vi "readQPD3axissignal.vi"(9 "error out":errorcluster, 10 "Samples per Channel":i32, 11 "task in":refnum<k21>) -> (1 "X mean":dbl, 2 "Y mean":dbl, 3 "Z mean":dbl)   [LabVIEW 2014]
doc: "Read QPD 3 axis signal according to the input DAQ task."
uses:
  <vilib>/Analysis/baseanly.llb/Mean (DBL).vi
  <vilib>/DAQmx/read.llb/DAQmx Read (Analog 2D DBL NChan NSamp).vi
  <vilib>/Analysis/NI_AALBase.lvlib
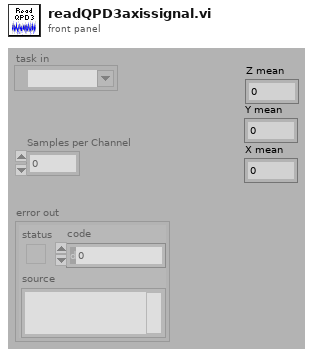
[diagram p1: front panel]
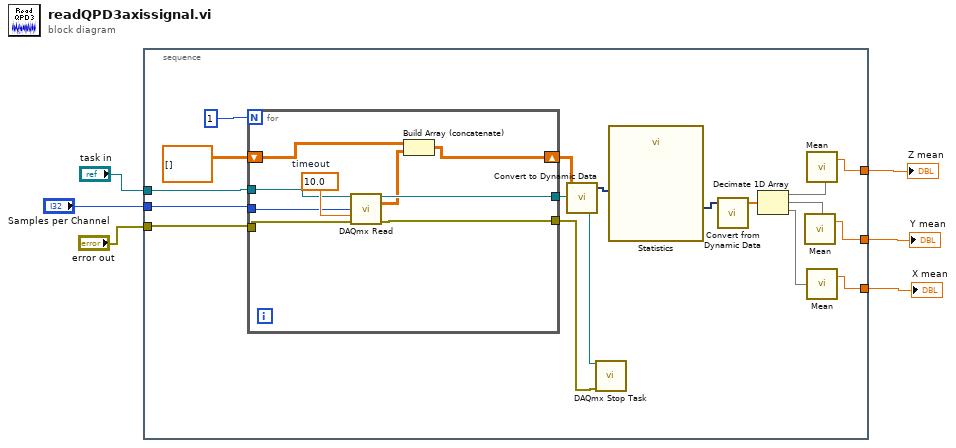
[diagram p0: block diagram]
diagram:
  n1 = stacked-sequence {
    tunnel: [w15] -> w6
    tunnel: [w14] -> w5
    tunnel: "task in" -> [w13]
    tunnel: "error out" -> [w12]
    tunnel: "Samples per Channel" -> [w11]
    tunnel: [w9] -> w4
    frame #0 {
      n2 = for {
        N: 1 -> [_]
        tunnel: [w32] -> w7
        tunnel: [w31] -> w8
        shift-right: [w29] -> w21
        shift-left: dbl[][] [] -> [w30]
        tunnel: w13 -> [w26]
        tunnel: w12 -> [w25]
        tunnel: w11 -> [w24]
        w28 = 10.0  # timeout
        n3 = call-poly <vilib>:"DAQmx Read.vi"("task/channels in"=w26, "number of samples per channel"=w24, "timeout"=w28, "error in"=w25) -> ("task out"=w32:refnum<k21>, "data"=w27:dbl[][], "error out"=w31:errorcluster)  [unwired: 9 out]
        n4 = Build Array (concatenate) "Build Array"(w30, w27) -> (w29:dbl[][])
      }
      n5 = call "Convert to Dynamic Data"("2D Array"=w21) -> ("Dynamic Data Type"=w20:dynamicdata)  [unwired: 3 out]
      n6 = call <vilib>:"DAQmx Stop Task.vi"("task/channels in"=w7, "error in"=w8) -> ()  [unwired: 14 out]
      n7 = call "Statistics"("Signals"=w20) -> ("Arithmetic Mean"=w17:dynamicdata)  [unwired: 1 in, 25 out]
      n8 = call "Convert from Dynamic Data"("Dynamic Data Type"=w17) -> ("Array"=w16:dbl[])  [unwired: 3 out]
      n9 = Decimate 1D Array(w16) -> (w19:dbl[], w18:dbl[], w10:dbl[])
      n10 = call-poly <vilib>:"Mean.vi"("X"=w18) -> ("mean"=w14:dbl)  [unwired: 1 out]
      n11 = call-poly <vilib>:"Mean.vi"("X"=w19) -> ("mean"=w15:dbl)  [unwired: 1 out]
      n12 = call-poly <vilib>:"Mean.vi"("X"=w10) -> ("mean"=w9:dbl)  [unwired: 1 out]
    }
  }
  "Z mean" <- w6
  "Y mean" <- w5
  "X mean" <- w4
